vi "Message.vi"(8 "error in (no error)":errorcluster, 10 "Message":string, 11 "abs_EventLog in":refnum<class "abs_EventLog.lvclass">) -> (0 "error out":errorcluster, 3 "abs_EventLog out":refnum<class "abs_EventLog.lvclass">)   [LabVIEW 2021, in "abs_EventLog.lvclass"]
uses:
  abs_EventLog.lvclass
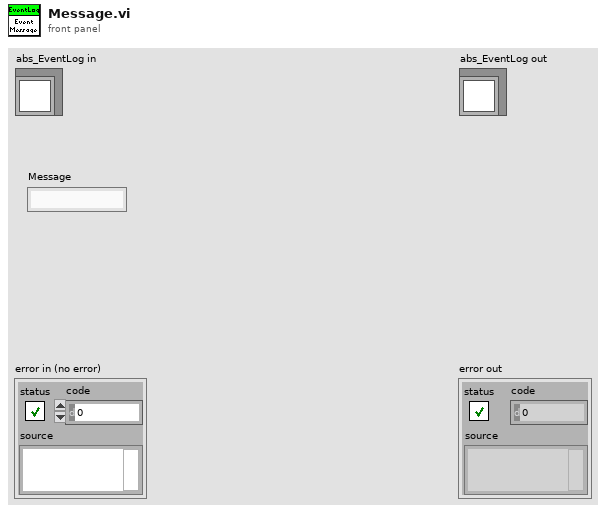
[diagram p1: front panel]
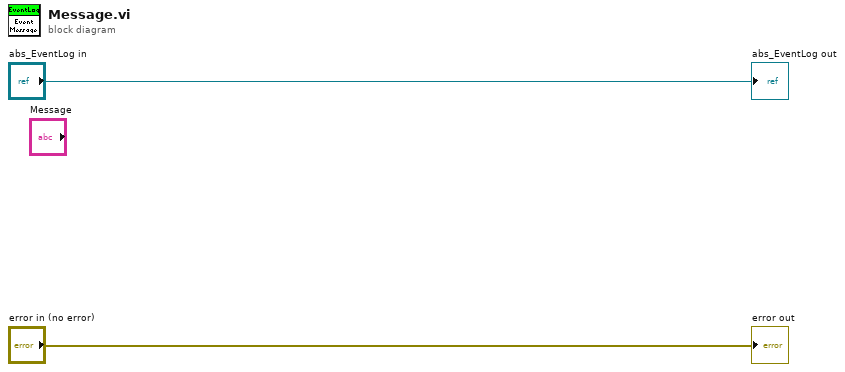
[diagram p0: block diagram]
diagram:
  "error out" <- "error in (no error)"
  "abs_EventLog out" <- "abs_EventLog in"
